vi "Read.vi"(8 "error in (no error)":errorcluster, 11 "ArduinoAI in":refnum<class "ArduinoAI.lvclass">) -> (0 "error out":errorcluster, 2 "data":dbl[][](array[numeric]), 3 "ArduinoAI out":refnum<class "ArduinoAI.lvclass">)   [LabVIEW 2020, in "ArduinoAI.lvclass"]
uses:
  ArduinoAI.lvclass
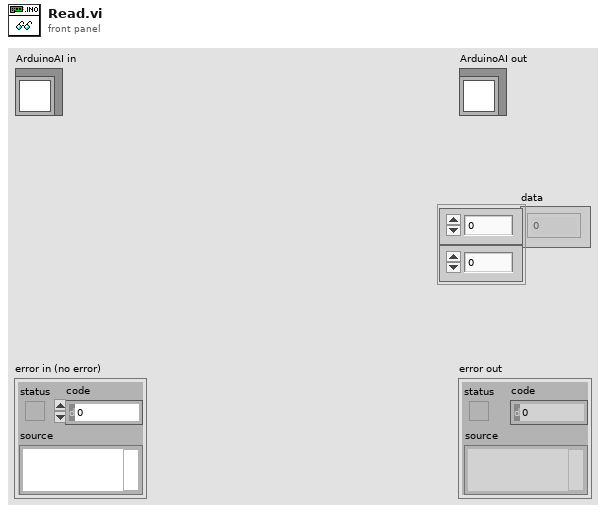
[diagram p1: front panel]
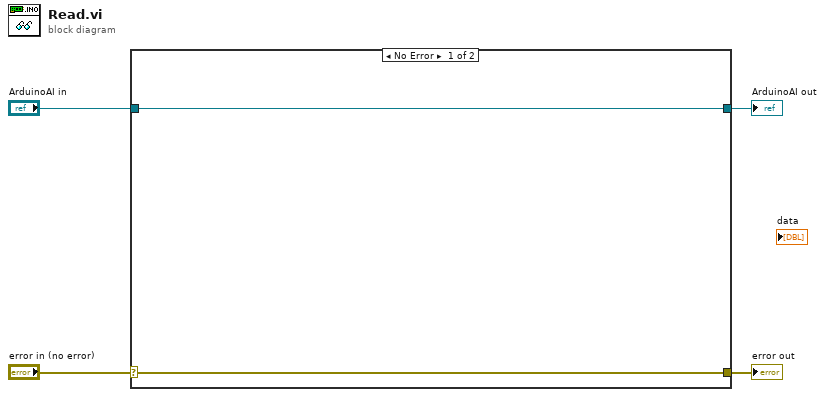
[diagram p0: block diagram]
diagram:
  n1 = case shown="No Error" "error in (no error)" {
    selector: "error in (no error)" -> [w5 w8]
    tunnel: [w5 w8] -> w3
    tunnel: [w6 w7] -> w1
    tunnel: "ArduinoAI in" -> [w6 w7]
    frame No Error {
    }
    frame Error {
    }
  }
  "error out" <- w3
  "ArduinoAI out" <- w1
